vi "Station_KVR.vi"() -> ()   [LabVIEW 2018]
uses:
  <vilib>/Instr/_visa.llb/VISA Configure Serial Port (Instr).vi
panel:
  out "Humidity":dbl(graph)
  out "Pressure":dbl(graph)
  out "Temperature":dbl(graph)
  out "Humidity":dbl
  out "Pressure":dbl
  out "Temperature":dbl
  out "Chaîne":string
  in  "Stop":bool
  in  "Nom de ressource VISA":refnum<visa-resource-name>
  # "1. Brancher la carte Arduino sur un port USB\n2. Choisir le port COM de la carte dans la liste déroulante \"Nom de ressource VISA\"\n3. Lancer le programme"
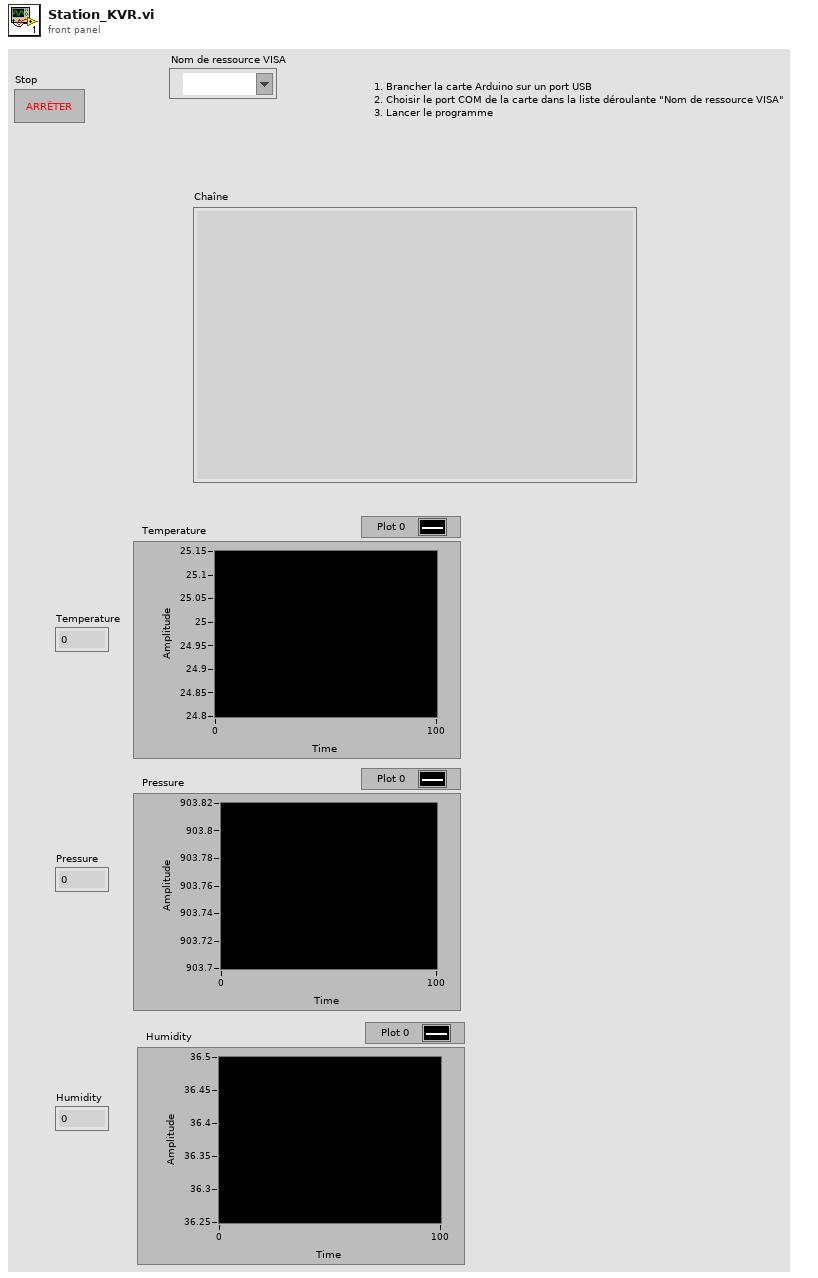
[diagram p1: front panel]
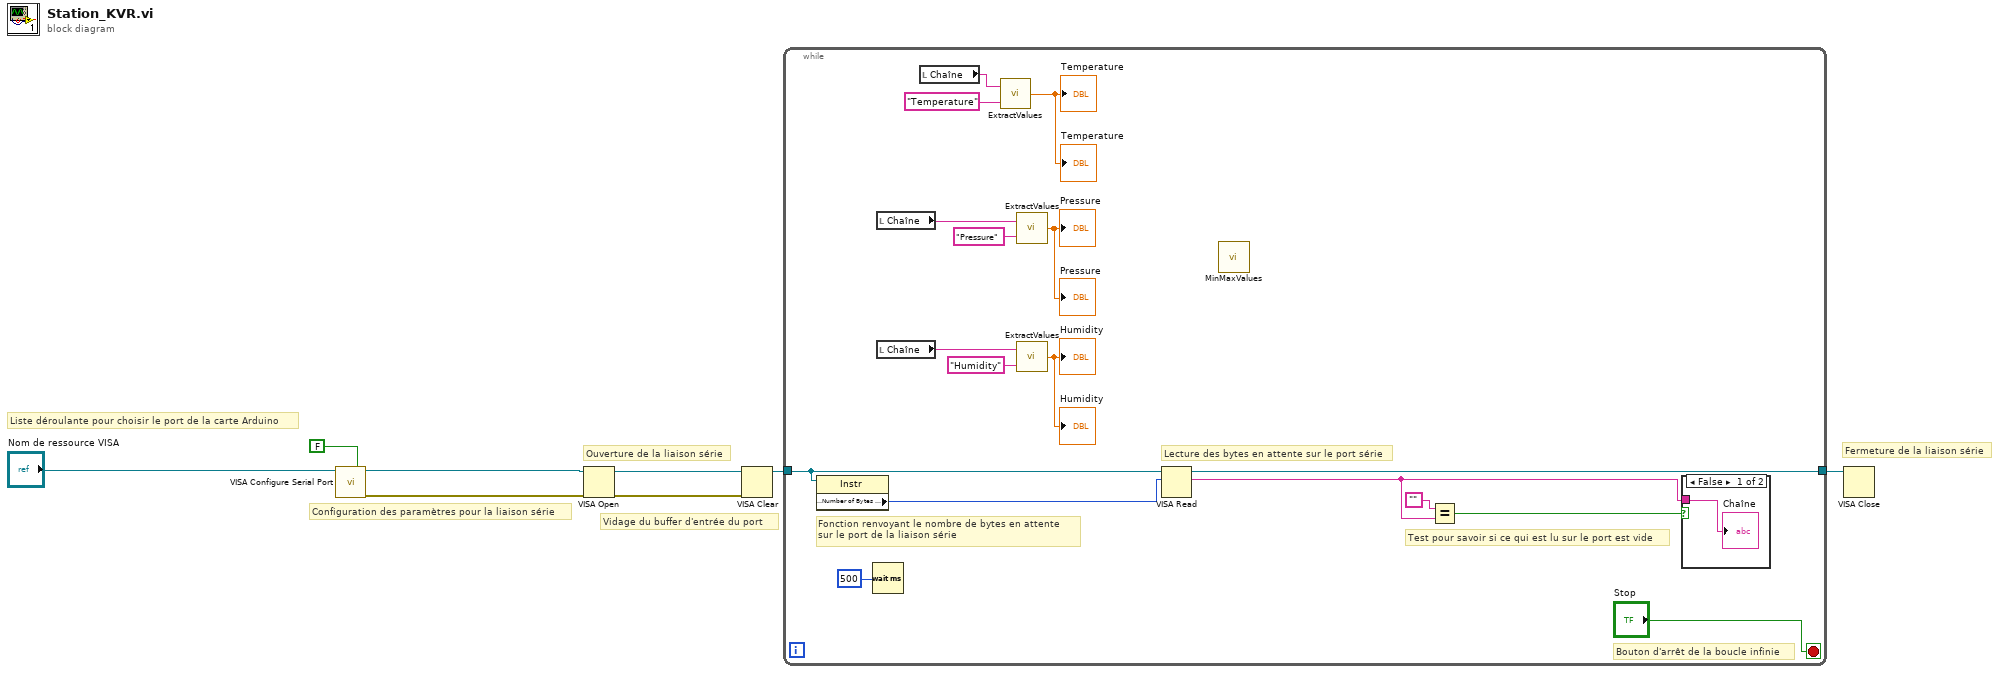
[diagram p0: block diagram]
diagram:
  # "Vidage du buffer d'entrée du port"
  # "Ouverture de la liaison série"
  # "Configuration des paramètres pour la liaison série"
  # "Liste déroulante pour choisir le port de la carte Arduino"
  # "Fermeture de la liaison série"
  n1 = call-poly "VISA Configure Serial Port"("VISA resource name"="Nom de ressource VISA", "Enable Termination\nChar (T)"=FALSE ("Enable Termination\nChar (T)")) -> ("VISA resource name out"=w5:refnum<visa-resource-name>, "error out"=w3:errorcluster)  [unwired: 12 in]
  n2 = VISA Open(error in (no error)=w3, VISA resource name=w5) -> (VISA resource name=w7:refnum<visa-resource-name>, error out=w2:errorcluster)  [unwired: 3 in]
  n3 = VISA Clear(VISA resource name=w7, error in (no error)=w2) -> (VISA resource name out=w6:refnum<visa-resource-name>)  [unwired: 1 out]
  n4 = while {
    tunnel: w6 -> [w24]
    tunnel: [w22] -> w1
    stop <- "Stop" stop-if-true
    # "Lecture des bytes en attente sur le port série"
    # "Fonction renvoyant le nombre de bytes en attente\nsur le port de la liaison série"
    # "Test pour savoir si ce qui est lu sur le port est vide"
    # "Bouton d'arrêt de la boucle infinie"
    n5 = property class="Instr"(reference=w24) -> ("Serial Settings:Number of Bytes at Serial Port"=w23:u32)  [unwired: 1 in, 2 out]
    n6 = Wait (ms)(milliseconds to wait=u32 500 ("attente (ms)")) -> ()  [unwired: 1 out]
    n7 = local read "Chaîne"() -> (w12:string)
    n8 = local read "Chaîne"() -> (w13:string)
    n9 = local read "Chaîne"() -> (w17:string)
    n10 = call "ExtractValues.vi"("Variable name"="Temperature", "Input String"=w17) -> ("Variable value"=→"Temperature" →"Temperature":dbl)
    n11 = call "ExtractValues.vi"("Variable name"="Pressure", "Input String"=w12) -> ("Variable value"=→"Pressure" →"Pressure":dbl)
    n12 = call "ExtractValues.vi"("Variable name"="Humidity", "Input String"=w13) -> ("Variable value"=→"Humidity" →"Humidity":dbl)
    n13 = VISA Read(VISA resource name=w24, byte count=w23) -> (VISA resource name out=w22:refnum<visa-resource-name>, read buffer=w18:string)  [unwired: 1 in, 2 out]
    n14 = call "MinMaxValues.vi"() -> ()  [unwired: 2 in, 2 out]
    n15 = Equal?(x="", y=w18) -> (x = y?=w19:bool)
    n16 = case shown="False" w19 {
      tunnel: w18 -> [w26 _]
      frame False {
        "Chaîne" <- w26
      }
      frame True {
      }
    }
  }
  n17 = VISA Close(VISA resource name=w1) -> ()  [unwired: 1 in, 1 out]
